vi "Return Delete Control Result.vi"(8 "error in (no error)":errorcluster, 10 "Label.Text":string, 11 "Delete Control (Console2API) in":refnum<class "Console Reply Delete Control.lvclass">) -> (0 "error out":errorcluster, 3 "Delete Control (Console2API) out":refnum<class "Console Reply Delete Control.lvclass">)   [LabVIEW 2015, in "Console Reply Delete Control.lvclass"]
uses:
  Console Reply Delete Control.lvclass
  Console Reply Delete Control.lvclass/Console Reply Delete Control.ctl
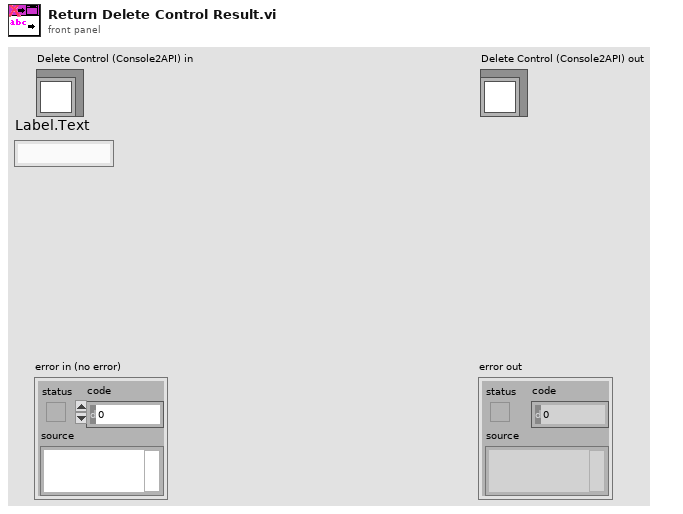
[diagram p1: front panel]
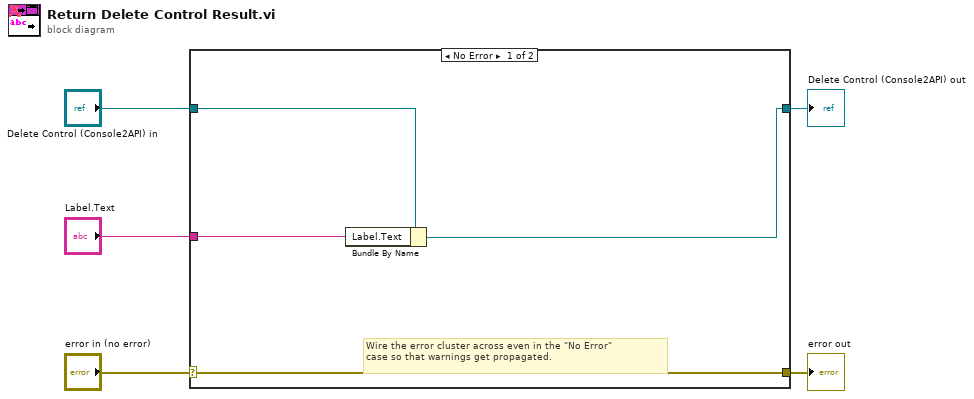
[diagram p0: block diagram]
diagram:
  n1 = case shown="No Error" "error in (no error)" {
    selector: "error in (no error)" -> [w9 w11]
    tunnel: [w9 w11] -> w4
    tunnel: [w6 w10] -> w2
    tunnel: "Delete Control (Console2API) in" -> [w8 w10]
    tunnel: "Label.Text" -> [w7 _]
    frame No Error {
      # "Wire the error cluster across even in the \"No Error\"\ncase so that warnings get propagated."
      n2 = Bundle By Name(cluster=w8, "Label.Text"=w7) -> (w6:refnum<class "Console Reply Delete Control.lvclass">)
    }
    frame Error {
    }
  }
  "error out" <- w4
  "Delete Control (Console2API) out" <- w2
